vi "CS++HBContent.vi"() -> (0 "CS++Classes & Messages":T1(array[cluster]))   [LabVIEW 2016]
doc: "Place actor and class constants that should be included included in an application on the blockdiagramm."
uses:
  <vilib>/ActorFramework/Message/Message.lvclass
  Packages/CSPP_DIM/Examples/CS++DIM-Client/CS++DIM-Client.lvclass
  C:/User/Brand/LVP/CSPP-Dev/Packages/CSPP_Core/Actors/CS++BaseActor/CS++BaseActor.lvclass
  Packages/CSPP_DIM/Examples/CS++DIM-Server/CS++DIM-Server.lvclass
  Packages/CSPP_Syslog/CS++Syslog.lvclass
  Packages/CSPP_OPCUA/CS++OPCUAInterface/CS++OPCUAInterface.lvclass
  Packages/CSPP_ObjectManager/CS++ObjectManager/CS++ObjectManager.lvclass
  Packages/BNT/BNT_DAQmx/BNT_DAQmx-MCSV/BNT_DAQmx-MCSV.lvclass
  Packages/BNT/BNT_DSCXYGraph/BNT_DSCXYGraph/BNT_DSCXYGraph.lvclass
  Packages/CSPP_Core/Actors/CS++BaseActor/CS++BaseActor.lvclass
panel:
  # "Place actor and class constants on the blockdiagramm."
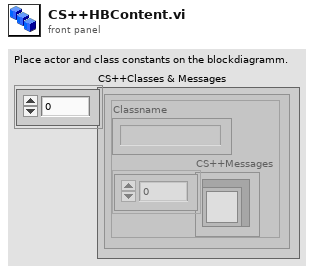
[diagram p1: front panel]
types:
  T1 = cluster{"Classname":string, "CS++Messages":refnum<class "Message.lvclass">[]}[]
  T2 = cluster{"class name":string, "CS++Messages":refnum<class "Message.lvclass">[]}
  T3 = cluster{"class name":string, "CS++Messages":refnum<class "Message.lvclass">[]}[]
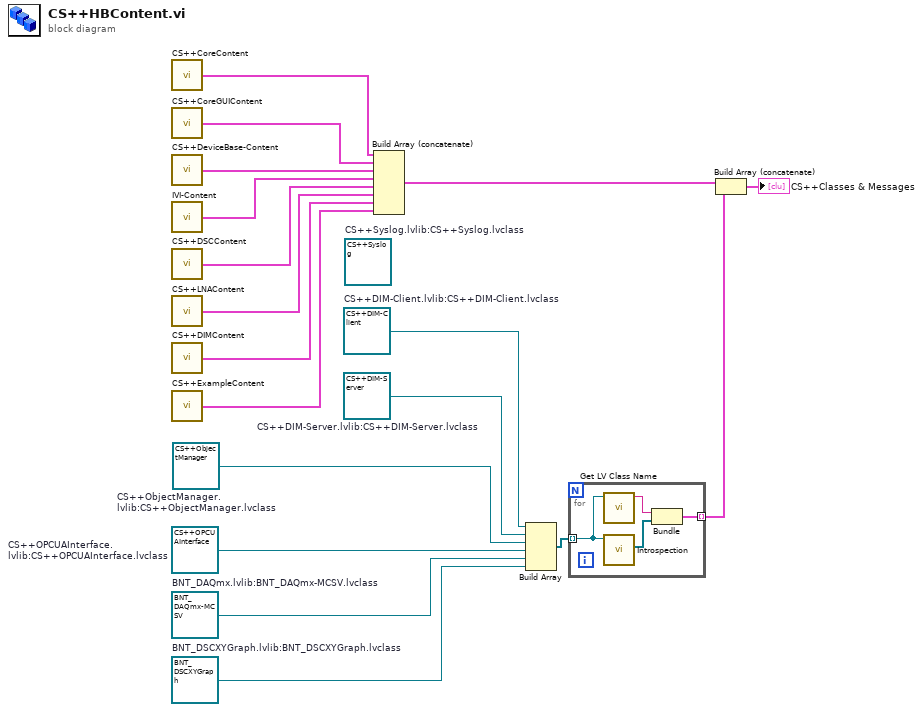
[diagram p0: block diagram]
diagram:
  w1 = refnum<class "BNT_DSCXYGraph.lvclass"> refnum  # BNT_DSCXYGraph.lvlib:BNT_DSCXYGraph.lvclass
  w2 = refnum<class "BNT_DAQmx-MCSV.lvclass"> refnum  # BNT_DAQmx.lvlib:BNT_DAQmx-MCSV.lvclass
  w5 = refnum<class "CS++ObjectManager.lvclass"> refnum  # CS++ObjectManager.lvlib:CS++ObjectManager.lvclass
  w10 = refnum<class "CS++OPCUAInterface.lvclass"> refnum  # CS++OPCUAInterface.lvlib:CS++OPCUAInterface.lvclass
  (unwired) refnum<class "CS++Syslog.lvclass"> refnum  # CS++Syslog.lvlib:CS++Syslog.lvclass
  w11 = refnum<class "CS++DIM-Server.lvclass"> refnum  # CS++DIM-Server.lvlib:CS++DIM-Server.lvclass
  w12 = refnum<class "CS++DIM-Client.lvclass"> refnum  # CS++DIM-Client.lvlib:CS++DIM-Client.lvclass
  n1 = call "CS++CoreContent.vi"() -> ("CS++Classes & Messages"=w4:T1)  [unwired: 1 in]
  n2 = call "CS++CoreGUIContent.vi"() -> ("CS++Classes & Messages"=w3:T1)  [unwired: 1 in]
  n3 = call "CS++DeviceBase-Content.vi"() -> ("CS++Classes & Messages"=w16:T1)  [unwired: 1 in]
  n4 = call "IVI-Content.vi"() -> ("CS++Classes & Messages"=w15:T1)  [unwired: 1 in]
  n5 = call "CS++DSCContent.vi"() -> ("CS++Classes & Messages"=w14:T1)  [unwired: 1 in]
  n6 = call "CS++LNAContent.vi"() -> ("CS++Classes & Messages"=w7:T1)  [unwired: 1 in]
  n7 = call "CS++DIMContent.vi"() -> ("CS++Classes & Messages"=w13:T1)  [unwired: 1 in]
  n8 = call "CS++ExampleContent.vi"() -> ("CS++Classes & Messages"=w6:T1)  [unwired: 1 in]
  n9 = Build Array (concatenate)(w4, w3, w16, w15, w14, w7, w13, w6) -> (w8:T1)
  n10 = Build Array(w12, w11, w5, w10, w2, w1) -> (w9:refnum<class "CS++BaseActor.lvclass">[])
  n11 = for {
    tunnel: w9 -> [w22] mode=indexing
    tunnel: [w19] -> w17 mode=indexing
    n12 = call <vilib>:"Get LV Class Name.vi"("object"=w22) -> ("class name"=w21:string)  [unwired: 9 in, 1 out]
    n13 = call "Introspection.vi"("CS++BaseActor in"=w22) -> ("CS++Messages"=w20:refnum<class "Message.lvclass">[])  [unwired: 8 in, 2 out]
    n14 = Bundle("class name"=w21, "CS++Messages"=w20) -> (w19:T2)  [unwired: 1 in]
  }
  n15 = Build Array (concatenate)(w8, w17) -> (→"CS++Classes & Messages":T3)
